vi "CLD 1 Elapsed Time Express Solution.vi"() -> ()   [LabVIEW 2009]
doc: "CLD-Übung 1\n\nDieses VI ist ein Aufrufer des Express-VIs. Das Express-VI ist ablaufinvariant. Seien Sie daher achtsam, wenn das Express-VI mehrfach in einem VI verwendet wird."
panel:
  out "Verstrichene Zeit (s)":dbl
  out "Zeit ist verstrichen":bool
  in  "Autom. zurücksetzen":bool
  in  "Zurücksetzen-Schaltfläche":bool
  in  "VI anhalten":bool
  out "Fehler (Ausgang)":errorcluster
  in  "Fehler (Eingang, kein Fehler)":errorcluster
  in  "Zielzeit (s)":dbl
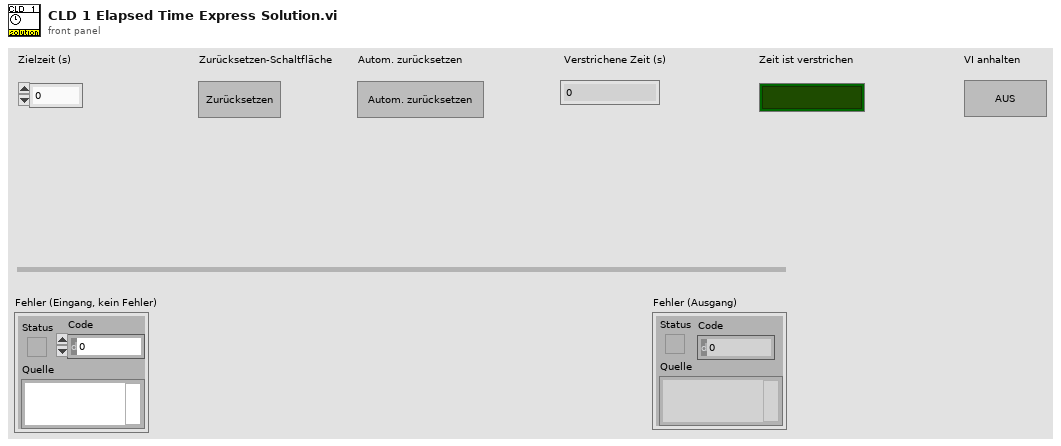
[diagram p1: front panel]
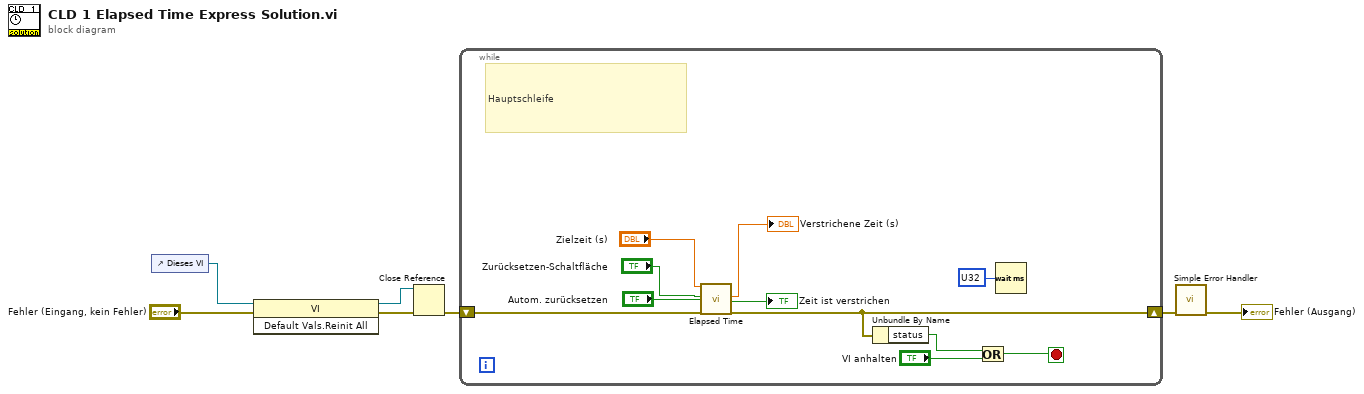
[diagram p0: block diagram]
diagram:
  n1 = control-ref of="Dieses VI"() -> (w4:refnum<vi>)
  n2 = invoke class="VI" method="Default Vals.Reinit All"(reference=w4, error in="Fehler (Eingang, kein Fehler)") -> (reference out=w2:refnum<vi>, error out=w5:errorcluster)  [unwired: 1 in, 1 out]
  n3 = Close Reference(reference=w2, error in (no error)=w5) -> (error out=w3:errorcluster)
  n4 = while {
    shift-right: [w12] -> w6
    shift-left: w3 -> [w16]
    stop <- w11 stop-if-true
    # "Hauptschleife"
    n5 = call "Elapsed Time"("Time Target (s)"="Zielzeit (s)", "Reset"="Zurücksetzen-Schaltfläche", "Auto Reset"="Autom. zurücksetzen", "error in (no error)"=w16) -> ("Elapsed Time (s)"=→"Verstrichene Zeit (s)":dbl, "Time has Elapsed"=→"Zeit ist verstrichen":bool, "error out"=w12:errorcluster)  [unwired: 8 in, 5 out]
    n6 = Unbundle By Name(w12) -> ("status"=w10:bool)
    n7 = Or(x=w10, y="VI anhalten") -> (x .or. y?=w11:bool)
    n8 = Wait (ms)(milliseconds to wait=u32 ? ("Zu wartende ms")) -> ()  [unwired: 1 out]
  }
  n9 = call <vilib>:"Simple Error Handler.vi"("error in (no error)"=w6) -> ("error out"=→"Fehler (Ausgang)":errorcluster)  [unwired: 4 in, 4 out]
